vi "Build.vi"(7 "CLI Output":refnum<class "CLI Output.lvclass">, 8 "error in (no error)":errorcluster, 9 "Library Description":string, 10 "NIPKG Inputs":T1, 11 "Installation Path":path=path "C:/LabVIEW Sources/PPLs/Windows/Release_32/blah.lvlibp") -> (0 "error out":errorcluster)   [LabVIEW 2019, in "NIPKG Packager.lvclass"]
uses:
  NIPKG Packager.lvclass
  CLI Output/CLI Output.lvclass
  NIPKG Inputs.ctl
  NIPKG Packager.lvclass/NIPKG Packager.ctl
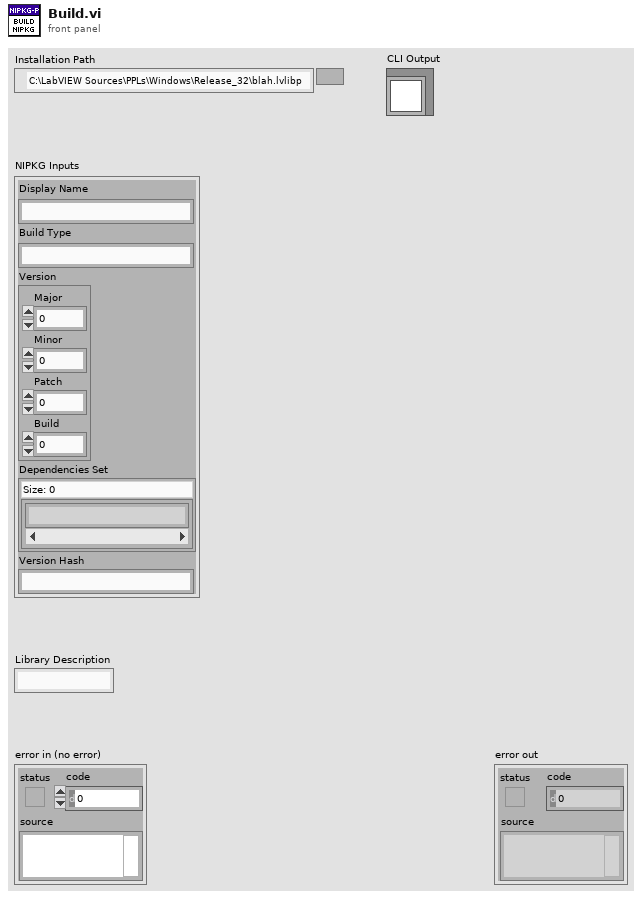
[diagram p1: front panel]
types:
  T1 = typedef "NIPKG Packager.lvclass/NIPKG Inputs.ctl" = cluster{"Display Name":string, "Build Type":string, "Version":cluster{"Major":i32, "Minor":i32, "Patch":i32, "Build":i32}, "Dependencies Set":set{string}, "Version Hash":string}
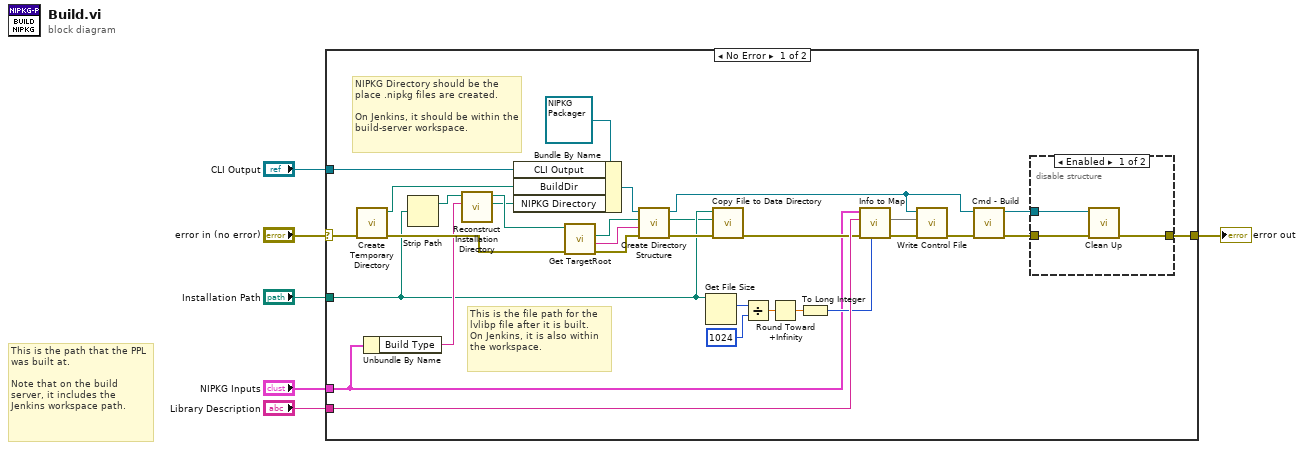
[diagram p0: block diagram]
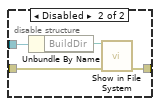
[diagram p2: hidden frame]
diagram:
  # "This is the path that the PPL was built at.\n\nNote that on the build server, it includes the Jenkins workspace path."
  n1 = case shown="No Error" "error in (no error)" {
    selector: "error in (no error)" -> [w34 w45]
    tunnel: [w25 w45] -> w5
    tunnel: "Installation Path" -> [w10 _]
    tunnel: "Library Description" -> [w35 _]
    tunnel: "CLI Output" -> [w12 _]
    tunnel: "NIPKG Inputs" -> [w11 _]
    frame No Error {
      # "This is the file path for the lvlibp file after it is built.\nOn Jenkins, it is also within the workspace."
      # "NIPKG Directory should be the place .nipkg files are created.\n\nOn Jenkins, it should be within the build-server workspace."
      n2 = call "Create Temporary Directory.vi"("error in"=w34) -> ("error out"=w33:errorcluster, "created path"=w32:path)  [unwired: 9 in]
      n3 = Unbundle By Name(w11) -> ("Build Type"=w15:string)
      n4 = Strip Path(path=w10) -> (stripped path=w9:path)  [unwired: 1 out]
      n5 = call "Reconstruct Installation Directory.vi"("Build Type"=w15, "Aliased Installation Path"=w9) -> ("NIPKG Directory"=w36:path, "Real Installation Path"=w37:path)  [unwired: 8 in]
      n6 = Bundle By Name(cluster=refnum<class "NIPKG Packager.lvclass"> refnum ("Packager in"), "CLI Output"=w12, "BuildDir"=w32, "NIPKG Directory"=w36) -> (w29:refnum<class "NIPKG Packager.lvclass">)
      n7 = call "Get TargetRoot.vi"("error in (no error)"=w33, "Installation Directory"=w37) -> ("error out"=w31:errorcluster, "Target Root Name"=w27:string, "Relative Path"=w28:path)  [unwired: 7 in]
      n8 = call "Create Directory Structure.vi"("error in (no error)"=w31, "TargetRoot Name"=w27, "Relative Directory Path"=w28, "NIPKG Packager in"=w29) -> ("error out"=w30:errorcluster, "Target File Directory"=w8:path, "NIPKG Packager out"=w7:refnum<class "NIPKG Packager.lvclass">)  [unwired: 4 in, 1 out]
      n9 = Get File Size(file=w10) -> (size (in bytes)=w21:i64)  [unwired: 1 in, 2 out]
      n10 = call "Copy File to Data Directory.vi"("error in (no error)"=w30, "Target File Directory"=w8, "Installation Path"=w10) -> ("error out"=w24:errorcluster)  [unwired: 8 in]
      n11 = Divide(x=w21, y=i64 1024) -> (x/y=w19:dbl)
      n12 = Round Toward +Infinity(x=w19) -> (ceil(x): smallest int >= x=w18:dbl)
      n13 = To Long Integer(number=w18) -> (32bit integer=w17:i32)
      n14 = call "Info to Map.vi"("File Size (kB)"=w17, "error in (no error)"=w24, "Library Description"=w35, "NIPKG Inputs"=w11) -> ("error out"=w23:errorcluster, "Map"=w22:map{string, string})  [unwired: 6 in]
      n15 = call "Write Control File.vi"("error in (no error)"=w23, "Map"=w22, "NIPKG Packager in"=w7) -> ("error out"=w26:errorcluster)  [unwired: 8 in]
      n16 = call "Cmd - Build.vi"("error in (no error)"=w26, "NIPKG Packager in"=w7) -> ("error out"=w14:errorcluster, "NIPKG Packager out"=w13:refnum<class "NIPKG Packager.lvclass">)  [unwired: 8 in]
      n17 = disable-structure shown="Enabled" {
        disable-tunnel: w13 -> [w40 w44]
        disable-tunnel: w14 -> [w39 w41]
        disable-tunnel: [w38 w42] -> w25
        frame Enabled {
          n18 = call "Clean Up.vi"("error in (no error)"=w39, "NIPKG Packager in"=w40) -> ("error out"=w38:errorcluster)  [unwired: 9 in]
        }
        frame Disabled {
          n19 = Unbundle By Name(w44) -> ("BuildDir"=w43:path)
          n20 = call <vilib>:"Show in File System.vi"("error in (no error)"=w41, "file or directory path"=w43) -> ("error out"=w42:errorcluster)  [unwired: 9 in]
        }
      }
    }
    frame Error {
    }
  }
  "error out" <- w5
